vi "Fifo Write.vi"(8 "error in (no error)":errorcluster, 10 "Data":u32[](array[numeric]), 11 "Refnum in":refnum<k20>) -> (0 "error out":errorcluster, 3 "Refnum out":refnum<k20>)   [LabVIEW 2013]
uses:
  <vilib>/rvi/interface/common/niFpgaWaitOnOcc.vi
  <vilib>/Utility/error.llb/Error Cluster From Error Code.vi
  <vilib>/rvi/errors/niLvFpgaAdjustHostInterfaceError.vi
  <vilib>/rvi/interface/nirviMethod/nirviMethod.xnode
  <vilib>/FPGAPlugInAG/Dynamic/niLvFpga_WriteFifo_Dynamic.vi
  <vilib>/rvi/errors/niLvFpgaMergeErrorWithErrorCode.vi
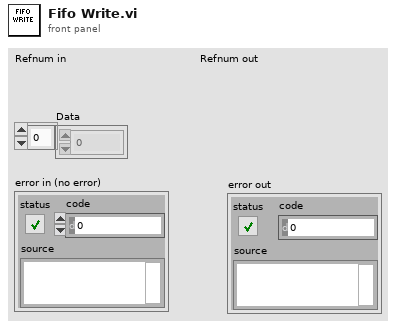
[diagram p1: front panel]
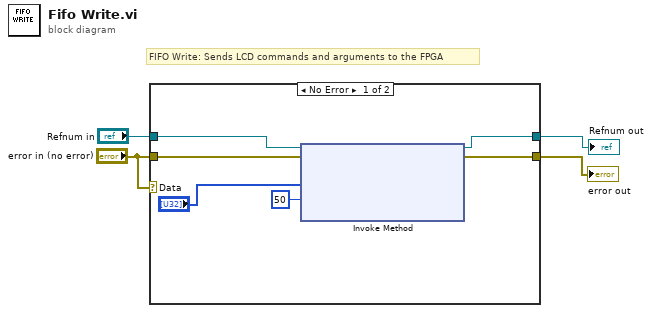
[diagram p0: block diagram]
diagram:
  # "FIFO Write: Sends LCD commands and arguments to the FPGA"
  n1 = case shown="No Error" "error in (no error)" {
    tunnel: [w10 w12] -> w4
    tunnel: "error in (no error)" -> [w9 w11]
    tunnel: "Refnum in" -> [w8 w12]
    tunnel: [w7 w11] -> w2
    frame No Error {
      n2 = xnode "Invoke Method"("FPGA VI Reference In"=w8, "error in"=w9, "Data"="Data", "Timeout (ms)"=50) -> ("FPGA VI Reference Out"=w10:refnum<k20>, "error out"=w7:errorcluster)  [unwired: 1 out]
    }
    frame Error {
    }
  }
  "Refnum out" <- w4
  "error out" <- w2
